vi "AuMT8852B Instrument Status Register Enable.vi"(5 "Flags":T1, 7 "Set/Get (Set)":enum16{"Set", "Get"}(ring), 8 "error in (no error)":errorcluster, 10 "Value (-1)":i32=-1, 11 "VISA session":refnum<visa-resource-name>) -> (0 "error out":errorcluster, 2 "error code":i32, 3 "VISA session out":refnum<visa-resource-name>, 4 "Flags out":T1, 6 "Value out":i32)   [LabVIEW 2017]
doc: "Anritsu MT8852B Bluetooth Tester\n\nIndicates which bits of the Instrument Status Register will cause a Service Request (SRQ). The value can be written as an integer (0-255), or as a cluster of flags.\n\nBit 2 - Script or test completion - this bit is cleared when a test or script has started and is set on its completion.\nBit 1 - Disconnect - this bit is cleared when a connection has been made and set when the EUT is disconnected..\nBit 0 (least significant bit) - Connection - this bit is set when a connection has been made and cleared when the connection no longer exists.\n\nINPUTS\nSet/Get - whether the values are being written to or read from the instrument.\nFlags - individual values to assign to the register.\nValue - integer value (0-255) to be written to the register. Leave this input unwired if you are using the Flags input.\n\nOUTPUTS\nFlags out - value of each bit in the register.\nValue out - integer value (0-255) of the register."
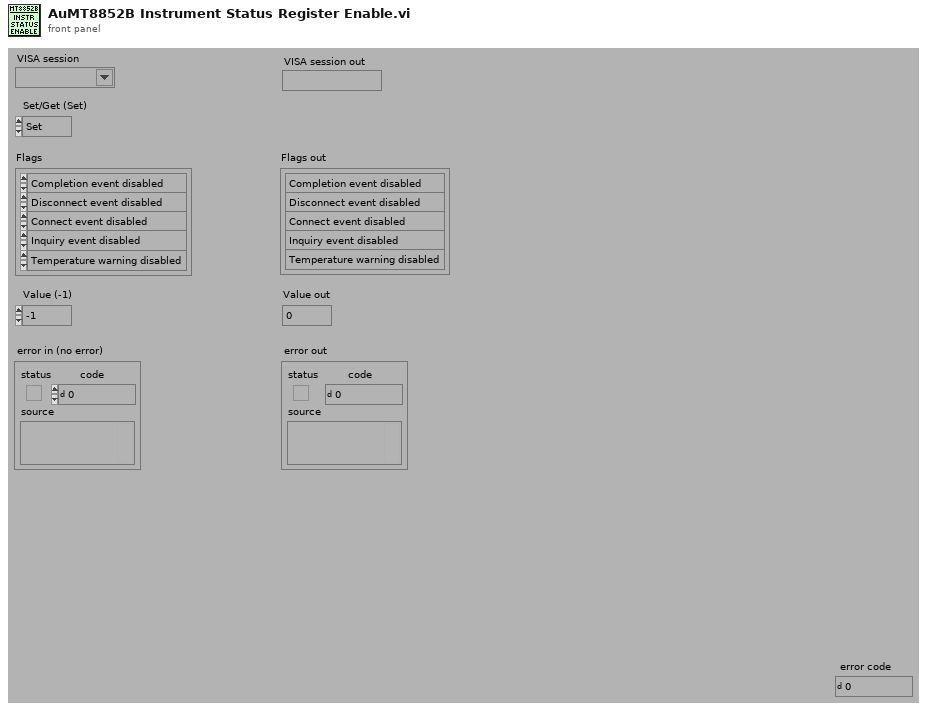
[diagram p1: front panel]
types:
  T1 = cluster{"Completion":enum16{"Completion event disabled", "Completion event enabled"}, "Disconnect":enum16{"Disconnect event disabled", "Disconnect event enabled"}, "Connect":enum16{"Connect event disabled", "Connect event enabled"}, "Inquiry":enum16{"Inquiry event disabled", "Inquiry event enabled"}, "Temperature":enum16{"Temperature warning disabled", "Temperature warning enabled"}}
  T2 = enum16{"Simulate", "Range check", "Cache", "Query instrument status"}
  T3 = cluster{"[0]":i16, "[1]":i16, "[2]":i16, "[3]":i16, "[4]":i16, "[5]":i16, "[6]":i16, "[7]":i16}
  T4 = enum16{"Connect event disabled", "Connect event enabled"}
  T5 = enum16{"Disconnect event disabled", "Disconnect event enabled"}
  T6 = enum16{"Completion event disabled", "Completion event enabled"}
  T7 = enum16{"Inquiry event disabled", "Inquiry event enabled"}
  T8 = enum16{"Temperature warning disabled", "Temperature warning enabled"}
  T9 = cluster{bool, bool, bool, bool, bool, bool, bool, bool}
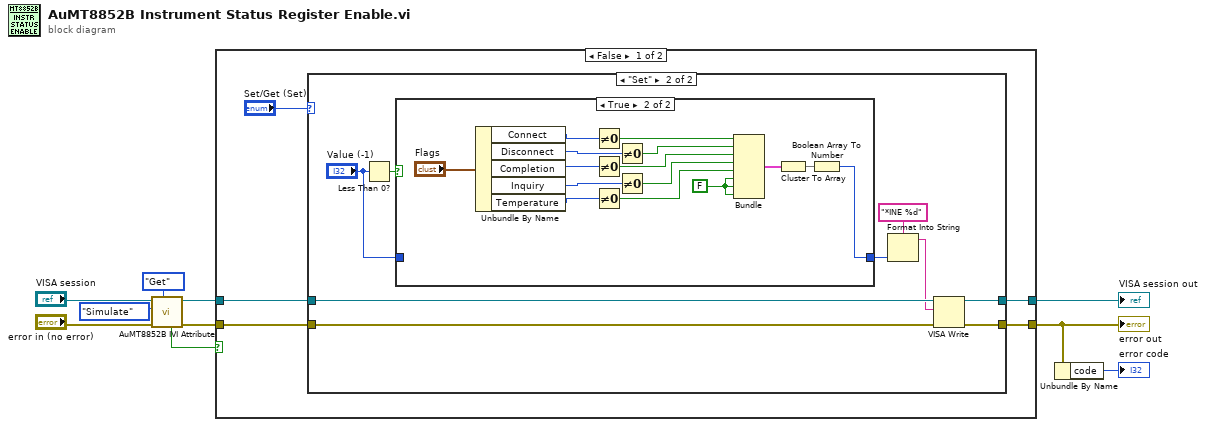
[diagram p0: block diagram]
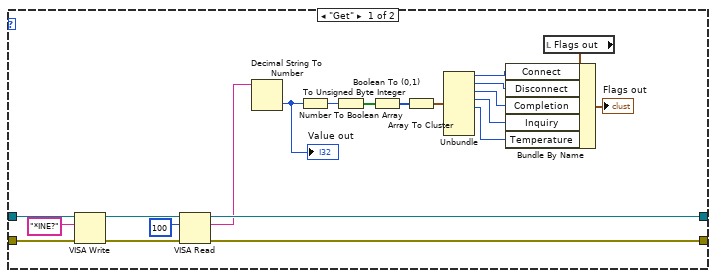
[diagram p2: hidden frame]
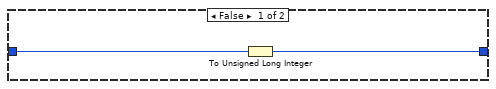
[diagram p3: hidden frame]
diagram:
  n1 = call <instrlib>:"AuMT8852B IVI Attribute.vi"("Set/Get (Set)"=enum16{"Set", "Get"}."Get", "error in (no error)"="error in (no error)", "Flag (Simulate)"=T2."Simulate", "VISA session"="VISA session") -> ("error out"=w6:errorcluster, "VISA session out"=w7:refnum<visa-resource-name>, "Value out"=w3:bool)  [unwired: 5 in]
  n2 = case shown="False" w3 {
    tunnel: [w12 w63] -> w1
    tunnel: [w13 w64] -> w8
    tunnel: w7 -> [w15 w64]
    tunnel: w6 -> [w14 w63]
    frame False {
      n3 = case shown="\"Set\"" "Set/Get (Set)" {
        tunnel: w15 -> [w36 w45]
        tunnel: w14 -> [w35 w44]
        tunnel: [w31 w41] -> w13
        tunnel: [w30 w40] -> w12
        frame "Get" {
          n4 = VISA Write(VISA resource name=w36, write buffer="*INE?" ("write buffer (\"\")"), error in (no error)=w35) -> (VISA resource name out=w33:refnum<visa-resource-name>, error out=w32:errorcluster)  [unwired: 1 out]
          n5 = VISA Read(VISA resource name=w33, byte count=u32 100 ("byte count (0)"), error in (no error)=w32) -> (VISA resource name out=w31:refnum<visa-resource-name>, read buffer=w28:string, error out=w30:errorcluster)  [unwired: 1 out]
          n6 = Decimal String To Number(string=w28) -> (number=w23:i32)  [unwired: 2 in, 1 out]
          "Value out" <- w23
          n7 = To Unsigned Byte Integer(number=w23) -> (unsigned 8bit integer=w24:u8)
          n8 = Number To Boolean Array(number=w24) -> (Boolean array=w25:bool[])
          n9 = Boolean To (0,1)(Boolean=w25) -> (0, 1=w26:i16[])
          n10 = Array To Cluster(array=w26) -> (cluster=w27:T3)
          n11 = Unbundle(w27) -> ("[0]"=w19:i16, "[1]"=w20:i16, "[2]"=w21:i16, "[3]"=w17:i16, "[4]"=w16:i16)  [unwired: 3 out]
          n12 = local read "Flags out"() -> (w22:T1)
          n13 = Bundle By Name(cluster=w22, "Connect"=w19, "Disconnect"=w20, "Completion"=w21, "Inquiry"=w17, "Temperature"=w16) -> (→"Flags out":T1)
        }
        frame "Set" {
          n14 = Less Than 0?(x="Value (-1)") -> (x < 0?=w38:bool)
          n15 = case shown="True" w38 {
            tunnel: [w46 w56] -> w42
            tunnel: "Value (-1)" -> [w47 _]
            frame False {
              n16 = To Unsigned Long Integer(number=w47) -> (unsigned 32bit integer=w46:u32)
            }
            frame True {
              w52 = FALSE
              n17 = Unbundle By Name("Flags") -> ("Connect"=w62:T4, "Disconnect"=w54:T5, "Completion"=w53:T6, "Inquiry"=w51:T7, "Temperature"=w50:T8)
              n18 = Not Equal To 0?(x=w62) -> (x != 0?=w61:bool)
              n19 = Not Equal To 0?(x=w53) -> (x != 0?=w59:bool)
              n20 = Not Equal To 0?(x=w50) -> (x != 0?=w48:bool)
              n21 = Not Equal To 0?(x=w54) -> (x != 0?=w60:bool)
              n22 = Not Equal To 0?(x=w51) -> (x != 0?=w49:bool)
              n23 = Bundle(w61, w60, w59, w49, w48, w52, w52, w52) -> (w58:T9)  [unwired: 1 in]
              n24 = Cluster To Array(cluster=w58) -> (array=w57:bool[])
              n25 = Boolean Array To Number(Boolean array=w57) -> (number=w56:u32)
            }
          }
          n26 = Format Into String(format string="*INE %d" ("Format String"), w42) -> (resulting string=w39:string)  [unwired: 2 in, 1 out]
          n27 = VISA Write(VISA resource name=w45, write buffer=w39, error in (no error)=w44) -> (VISA resource name out=w41:refnum<visa-resource-name>, error out=w40:errorcluster)  [unwired: 1 out]
        }
      }
    }
    frame True {
    }
  }
  "error out" <- w1
  "VISA session out" <- w8
  n28 = Unbundle By Name(w1) -> ("code"=→"error code":i32)
